vi "update_message.vi"(7 "error in (no error)":errorcluster, 10 "Cluster":T1) -> (0 "error out":errorcluster, 3 "Screen":string)   [LabVIEW 2017]
uses:
  controls/UpdateMessageCtl.ctl
  controls/UpdateMessageCmd.ctl
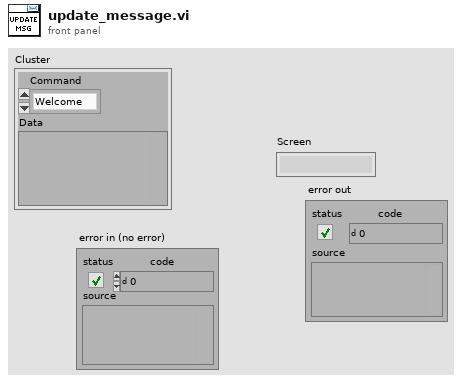
[diagram p1: front panel]
types:
  T1 = typedef "UpdateMessageCtl.ctl" = cluster{"Command":T2, "Data":variant}
  T2 = typedef "UpdateMessageCmd.ctl" = enum16{"Welcome"}
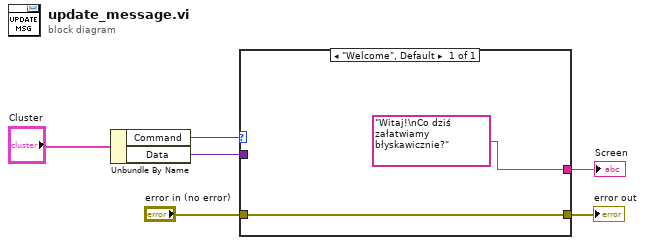
[diagram p0: block diagram]
diagram:
  n1 = Unbundle By Name("Cluster") -> ("Command"=w6:T2, "Data"=w5:variant)
  n2 = case shown="\"Welcome\", Default" w6 {
    tunnel: w5 -> [_]
    tunnel: "error in (no error)" -> [w8]
    tunnel: [w8] -> w3
    tunnel: ["Witaj!\nCo dziś załatwiamy błyskawicznie?"] -> w2
    frame "Welcome", Default {
    }
  }
  "error out" <- w3
  "Screen" <- w2
